vi "Agilent 681x Acquire Current Measurement.vi"() -> ()   [LabVIEW 2019]
doc: "Shows how to acquire a current measurement."
uses:
  <instrlib>/Agilent 681x Series/Public/Data/Read Single Measurement (Current).vi
  <instrlib>/Agilent 681x Series/Agilent 681x Series.lvlib
panel:
  in  "Sample Spacing (25 us)":dbl=2.5e-05 format="%^.2g"
  in  "Sense Source (0: Internal)":u16(ring) items=["Internal", "External"]
  in  "Output Frequency (60 Hz)":dbl=60.0 format="%#.4g"
  in  "Voltage Amplitude (1.0 V)":dbl=1.0 format="%#.4g"
  in  "Relative Trigger Samples (0)":i32
  in  "Output Waveform Type (0: Sinusoid)":u16(ring) items=["Sinusoid", "Square", "Clipped Sinusoid", "User Specified"]
  out "Peak Current":dbl
  out "AC + DC RMS Current":dbl
  out "AC RMS Current":dbl
  out "DC Current":dbl
  in  "Maximum Time (10000 ms)":i32=10000
  in  "User-Specified Output Waveform Name":string
  in  "Serial Configuration":T1={"Baud Rate"=9600, "Parity"=0, "Data Bits"=7} {"Data Bits" items=["7"=7, "8"=8]; "Parity" items=["None", "Odd", "Even", "Mark", "Space"]; "Baud Rate" items=["300"=300, "600"=600, "1200"=1200, "2400"=2400, "4800"=4800, "9600"=9600]}
  in  "VISA resource name":refnum<visa-resource-name>
  # "(c) 2008-2021 National Instruments Corp.  ALL RIGHTS RESERVED."
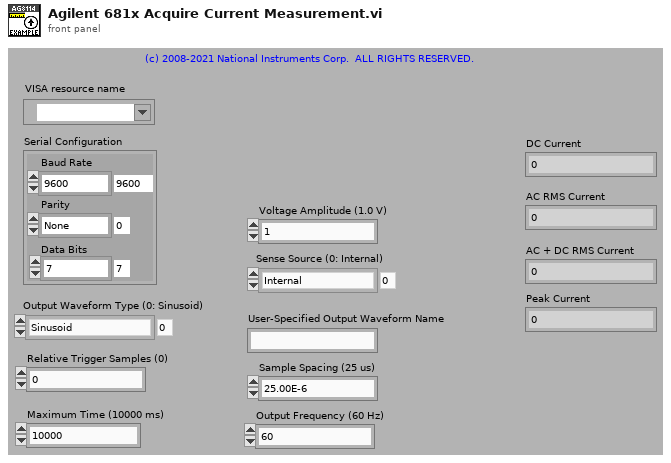
[diagram p1: front panel]
types:
  T1 = cluster{"Baud Rate":u32, "Parity":u16, "Data Bits":u16}
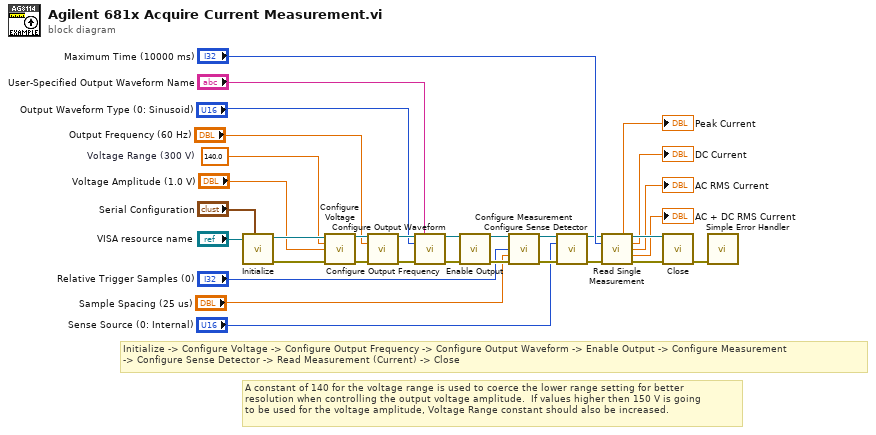
[diagram p0: block diagram]
diagram:
  w28 = 140.0  # Voltage Range (300 V)
  # "Initialize -> Configure Voltage -> Configure Output Frequency -> Configure Output Waveform -> Enable Output -> Configure Measurement\n-> Configure Sense Detector -> Read Measurement (Current) -> Close"
  # "A constant of 140 for the voltage range is used to coerce the lower range setting for better\nresolution when controlling the output voltage amplitude.  If values higher then 150 V is going\nto be used for the voltage amplitude, Voltage Range constant should also be increased."
  n1 = call <instrlib>:"Initialize.vi"("Serial Configuration"="Serial Configuration", "VISA resource name"="VISA resource name") -> ("error out"=w29:errorcluster, "VISA resource name out"=w30:refnum<visa-resource-name>)  [unwired: 8 in]
  n2 = call <instrlib>:"Configure Voltage.vi"("VISA resource name"=w30, "Voltage Range (300 V)"=w28, "Voltage Amplitude (1.0 V)"="Voltage Amplitude (1.0 V)", "error in (no error)"=w29) -> ("VISA resource name out"=w14:refnum<visa-resource-name>, "error out"=w15:errorcluster)  [unwired: 10 in]
  n3 = call <instrlib>:"Configure Output Frequency.vi"("VISA resource name"=w14, "Output Frequency (60 Hz)"="Output Frequency (60 Hz)", "error in (no error)"=w15) -> ("VISA resource name out"=w24:refnum<visa-resource-name>, "error out"=w25:errorcluster)  [unwired: 11 in]
  n4 = call <instrlib>:"Configure Output Waveform.vi"("VISA resource name"=w24, "User-Specified Output Waveform Name"="User-Specified Output Waveform Name", "Output Waveform Type (0: Sinusoid)"="Output Waveform Type (0: Sinusoid)", "error in (no error)"=w25) -> ("VISA resource name out"=w26:refnum<visa-resource-name>, "error out"=w27:errorcluster)  [unwired: 10 in]
  n5 = call <instrlib>:"Enable Output.vi"("VISA resource name"=w26, "error in (no error)"=w27) -> ("VISA resource name out"=w22:refnum<visa-resource-name>, "error out"=w21:errorcluster)  [unwired: 12 in]
  n6 = call <instrlib>:"Configure Measurement.vi"("VISA resource name"=w22, "Relative Trigger Samples (0)"="Relative Trigger Samples (0)", "Sample Spacing (25 us)"="Sample Spacing (25 us)", "error in (no error)"=w21) -> ("VISA resource name out"=w20:refnum<visa-resource-name>, "error out"=w19:errorcluster)  [unwired: 10 in]
  n7 = call <instrlib>:"Configure Sense Detector.vi"("VISA resource name"=w20, "Sense Source (0: Internal)"="Sense Source (0: Internal)", "error in (no error)"=w19) -> ("VISA resource name out"=w16:refnum<visa-resource-name>, "error out"=w17:errorcluster)  [unwired: 11 in]
  n8 = call-poly <instrlib>:"Read Single Measurement.vi"("VISA resource name"=w16, "Maximum Time (10000 ms)"="Maximum Time (10000 ms)", "error in (no error)"=w17) -> ("Peak Current"=→"Peak Current":dbl, "VISA resource name out"=w12:refnum<visa-resource-name>, "DC Current"=→"DC Current":dbl, "AC RMS Current"=→"AC RMS Current":dbl, "AC + DC RMS Current"=→"AC + DC RMS Current":dbl, "error out"=w13:errorcluster)  [unwired: 7 in]
  n9 = call <instrlib>:"Close.vi"("error in (no error)"=w13, "VISA resource name"=w12) -> ("error out"=w11:errorcluster)  [unwired: 9 in]
  n10 = call <vilib>:"Simple Error Handler.vi"("error in (no error)"=w11) -> ()  [unwired: 4 in, 5 out]
